vi "ESN_evaluateByMSE(Array).vi"(8 "error in (no error)":errorcluster, 10 "desired output":dbl[](array[numeric]), 11 "output":dbl[](array[numeric])) -> (0 "error out":errorcluster, 3 "MSE":dbl)   [LabVIEW 2017]
uses:
  <vilib>/Analysis/NI_AALPro.lvlib
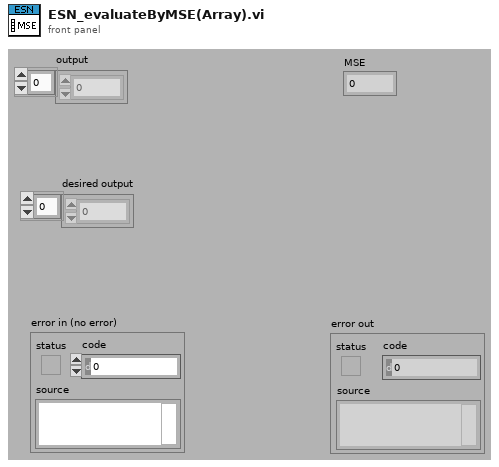
[diagram p1: front panel]
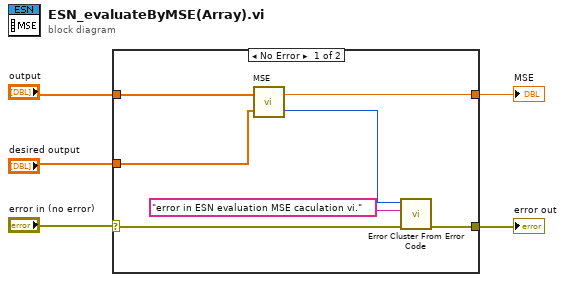
[diagram p0: block diagram]
diagram:
  n1 = case shown="No Error" "error in (no error)" {
    selector: "error in (no error)" -> [w11 w13]
    tunnel: "output" -> [w8 _]
    tunnel: "desired output" -> [w7 _]
    tunnel: [w6 _] -> w3
    tunnel: [w10 w13] -> w1
    frame No Error {
      n2 = call <vilib>:"MSE.vi"("X Values"=w7, "Y Values"=w8) -> ("error"=w12:i32, "mse"=w6:dbl)
      n3 = call <vilib>:"Error Cluster From Error Code.vi"("error in (no error)"=w11, "error message (\"\")"="error in ESN evaluation MSE caculation vi." ("source messages"), "error code (0)"=w12) -> ("error out"=w10:errorcluster)  [unwired: 6 in]
    }
    frame Error {
    }
  }
  "MSE" <- w3
  "error out" <- w1
